vi "SCALERS_DELAY.vi"(8 "error out 2":errorcluster, 10 "Ventana 2":u32, 11 "ftHandle_out 2":u32) -> (0 "error out":errorcluster, 3 "ftHandle_out":u32)   [LabVIEW 2019]
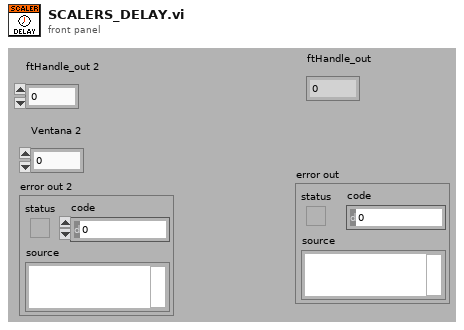
[diagram p1: front panel]
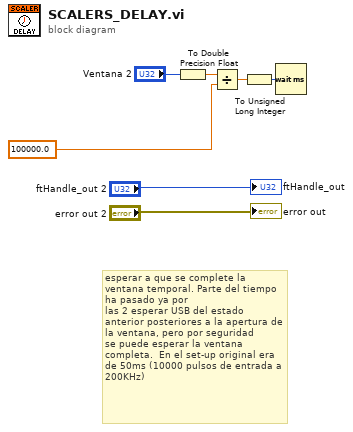
[diagram p0: block diagram]
diagram:
  # "esperar a que se complete la ventana temporal. Parte del tiempo ha pasado ya por\nlas 2 esperar USB del estado anterior posteriores a la apertura de la ventana, pero por seguridad\nse puede esperar la ventana completa.  En el set-up original era de 50ms (10000 pulsos de entrada a 200KHz)"
  n1 = To Double Precision Float(number="Ventana 2") -> (double precision float=w3:dbl)
  n2 = Divide(x=w3, y=100000.0 ("Ventana")) -> (x/y=w4:dbl)
  n3 = To Unsigned Long Integer(number=w4) -> (unsigned 32bit integer=w2:u32)
  n4 = Wait (ms)(milliseconds to wait=w2) -> ()  [unwired: 1 out]
  "error out" <- "error out 2"
  "ftHandle_out" <- "ftHandle_out 2"
